vi "myRIO_BRig_Host_TCP_parseCmd_block.vi"(10 "input_countCmd":i32, 11 "input_strCmd":string) -> (0 "output_L_or_R":i32, 2 "output_iBlock_num":i32, 3 "output_iBlock_str":string)   [LabVIEW 2014]
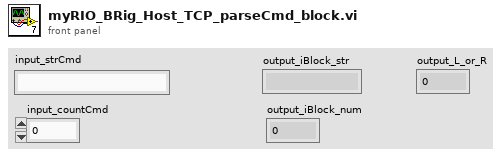
[diagram p1: front panel]
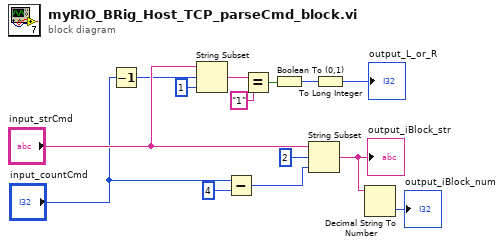
[diagram p0: block diagram]
diagram:
  n1 = Decrement(x="input_countCmd") -> (x-1=w12:i32)
  n2 = String Subset(string="input_strCmd", offset (0)=w12, length (rest)=1 ("length (rest)")) -> (substring=w11:string)
  n3 = Subtract(x="input_countCmd", y=4) -> (x-y=w3:i32)
  n4 = Equal?(x=w11, y="1") -> (x = y?=w9:bool)
  n5 = Boolean To (0,1)(Boolean=w9) -> (0, 1=w8:i16)
  n6 = String Subset(string="input_strCmd", offset (0)=2, length (rest)=w3) -> (substring=w14:string)
  "output_iBlock_str" <- w14
  n7 = To Long Integer(number=w8) -> (32bit integer=→"output_L_or_R":i32)
  n8 = Decimal String To Number(string=w14) -> (number=→"output_iBlock_num":i32)  [unwired: 2 in, 1 out]
